vi "write keyword - float.vi"(8 "error in (no error)":errorcluster, 9 "Value":dbl, 10 "keyword":string, 11 "Simulated_Header in":refnum<class "Simulated_Header.lvclass">) -> (0 "error out":errorcluster, 3 "Simulated_Header out":refnum<class "Simulated_Header.lvclass">)   [LabVIEW 2018, in "Simulated_Header.lvclass"]
uses:
  Simulated_Header.lvclass
  Simulated_Header.lvclass/Simulated_Header.ctl
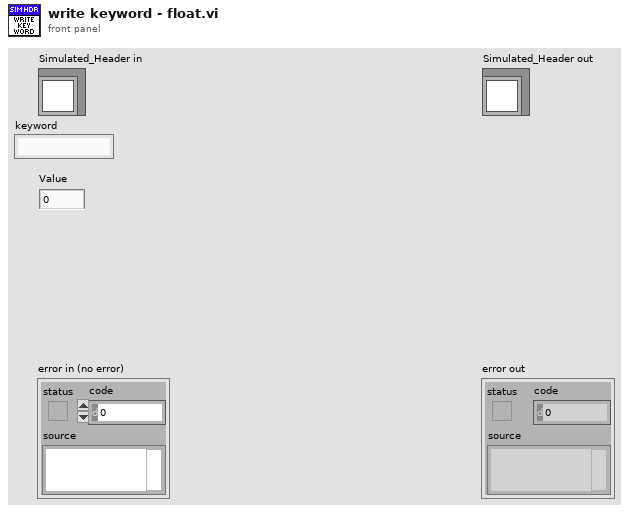
[diagram p1: front panel]
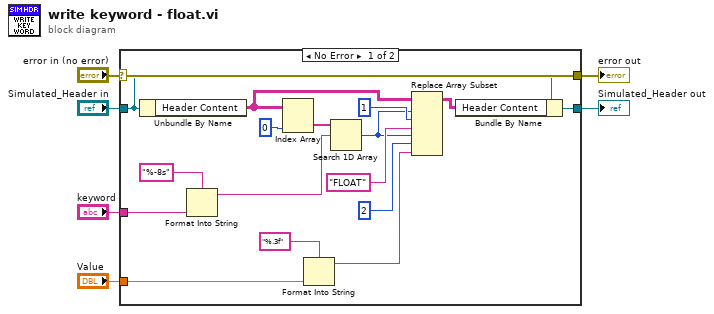
[diagram p0: block diagram]
diagram:
  n1 = case shown="No Error" "error in (no error)" {
    selector: "error in (no error)" -> [w23 w25]
    tunnel: [w23 w25] -> w5
    tunnel: [w17 w24] -> w3
    tunnel: "Simulated_Header in" -> [w18 w24]
    tunnel: "keyword" -> [w14 _]
    tunnel: "Value" -> [w9 _]
    frame No Error {
      n2 = Unbundle By Name(w18) -> ("Header Content"=w20:string[][])
      n3 = Format Into String(format string="%-8s", w14) -> (resulting string=w13:string)  [unwired: 2 in, 1 out]
      n4 = Index Array(array=w20, index (col)=0 ("disabled index (col)")) -> (element=w21:string[])  [unwired: 1 in]
      n5 = Format Into String(format string="%.3f", w9) -> (resulting string=w7:string)  [unwired: 2 in, 1 out]
      n6 = Search 1D Array(1D array=w21, element=w13) -> (index of element=w11:i32)  [unwired: 1 in]
      n7 = Replace Array Subset(array=w20, new element #1="FLOAT" ("new element/subarray"), index (row) #1=w11, index (col) #1=1 ("disabled index (col)"), new element #2=w7, index (row) #2=w11, index (col) #2=2 ("disabled index (col)")) -> (w16:string[][])
      n8 = Bundle By Name(cluster=w18, "Header Content"=w16) -> (w17:refnum<class "Simulated_Header.lvclass">)
    }
    frame Error {
    }
  }
  "error out" <- w5
  "Simulated_Header out" <- w3
